vi "Main DAQ Control.vi"() -> ()   [LabVIEW 2012]
uses:
  XControl.xctl
  <vilib>/UeiDaq/UeiDaqCreateDOSession.vi
  <vilib>/UeiDaq/UeiDaqConfigureTimingForSimpleIO.vi
  <vilib>/UeiDaq/UeiDaqWriteOneDigitalScanUInt16.vi
  <vilib>/UeiDaq/UeiDaqWriteDigitalDataUInt16.vi
  <resource>/objmgr/UeiDaq.rc
panel:
  out "Status Indicator":bool[][](array[boolean])
  out "Total Step":u64
  in  "Original Timing Signal (Timing Sequence from Timing File, adjustable on spot)":i16[][](array[numeric])=[[0, 0, 0, 0, 0, 0, 0, 0, 0, 0, 0, 0, 0, 0, 0, 0, 0, 0, 0, 0]] format="%b"
  in  "Digital Output Group 8":T1(xcontrol)
  in  "Digital Output Group 7":T1(xcontrol)
  in  "Group 6":T1(xcontrol)
  in  "Group 5":T1(xcontrol)
  in  "Group 4":T1(xcontrol)
  in  "Group 3":T1(xcontrol)
  in  "Group 2":T1(xcontrol)
  in  "Digital Output Group 1":T1(xcontrol) caption="Group 1"
  out "Running":bool
  in  "DIO Port":string="pwrdaq://Dev0/Do0:2"
  in  "stop":bool
  out "Loop Count":i32
  in  "Loop":bool
  out "Parsed File Location":path
  in  "All Low":bool
  in  "Run":bool
  in  "Timing Array":i32[](array[numeric])=[0, 0, 0, 0, 0, 0, 0, 0, 0, 0, 0, 0, 0, 0, 0, 0, 0, 0, 0, 0] caption="Timing Array (Time Duration for each signal)"
  out "Modified Timing Signal":u16[][](array[numeric]) caption="Modified Timing Signal (after adjustment from I/O channel panel)" format="%b"
  in  "Compile":bool
  in  "GPIB 2":string
  in  "GPIB 1":string
  out "Channel Names":string[](array[string])
  in  "Channel Number":u16
  in  "Load":bool
  in  "Timing File":path
  in  "Perl Parser":path=path "C:/Labview/Parser File/parse-timing.pl"
  # "(Use Do0:5 for DIO0-DIO5, 6ch,  Do0;5 for DIO0 and DIO5, 2ch)"
  # "Control Panel"
  # "(pwrdaq://Dev0 for real I/O; simu://Dev2 for simulated DAQ card)"
  # "I/O Channel"
  # "1"
  # "2"
  # "3"
  # "4"
  # "5"
  # "6"
  # "7"
  # "8"
  # "9"
  # "10"
  # "11"
  # "12"
  # "13"
  # "14"
  # "15"
  # "16"
  # "1"
  # "2"
  # "Group1"
  # "3"
  # "Group2"
  # "4"
  # "Group3"
  # "5"
  # "Group4"
  # "6"
  # "7"
  # "Group5"
  # "8"
  # "Group6"
  # "(Currently, When \"STOP\" is pressed, the status remain in the final state)"
  # "Status Panel"
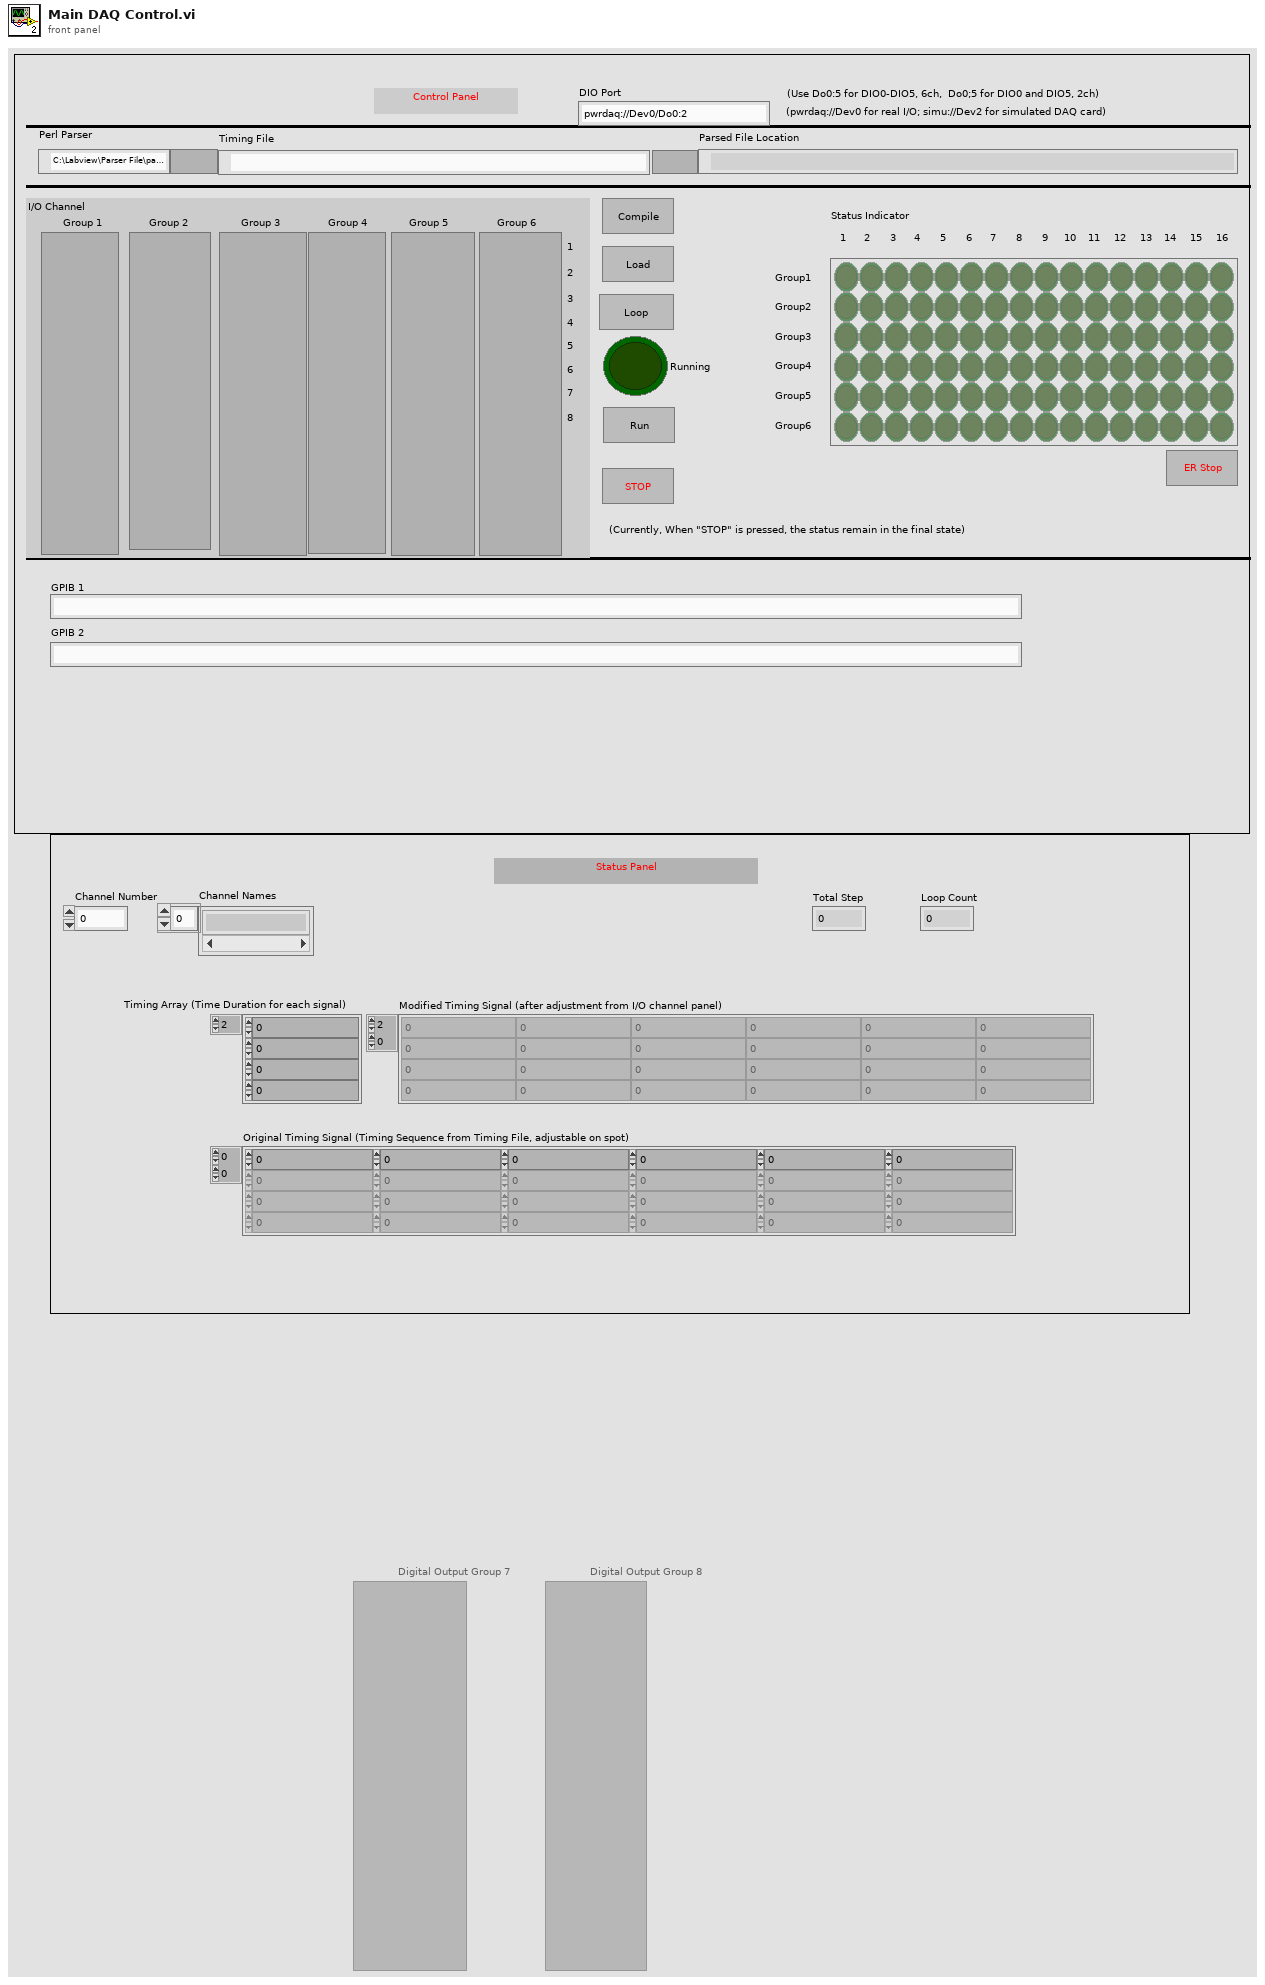
[diagram p1: front panel]
types:
  T1 = cluster{"Channel 1":u8, "Enable":bool, "Main Switch":u8, "Channel 2":u8, "Channel 3":u8, "Channel 4":u8, "Channel 1":u8, "Channel 5":u8, "Channel 6":u8, "Channel 7":u8, "Channel 8":u8, "Channel 9":u8, "Channel 10":u8, "Channel 11":u8, "Channel 1":u8, "Channel 12":u8, "Channel 13":u8, "Channel 14":u8}
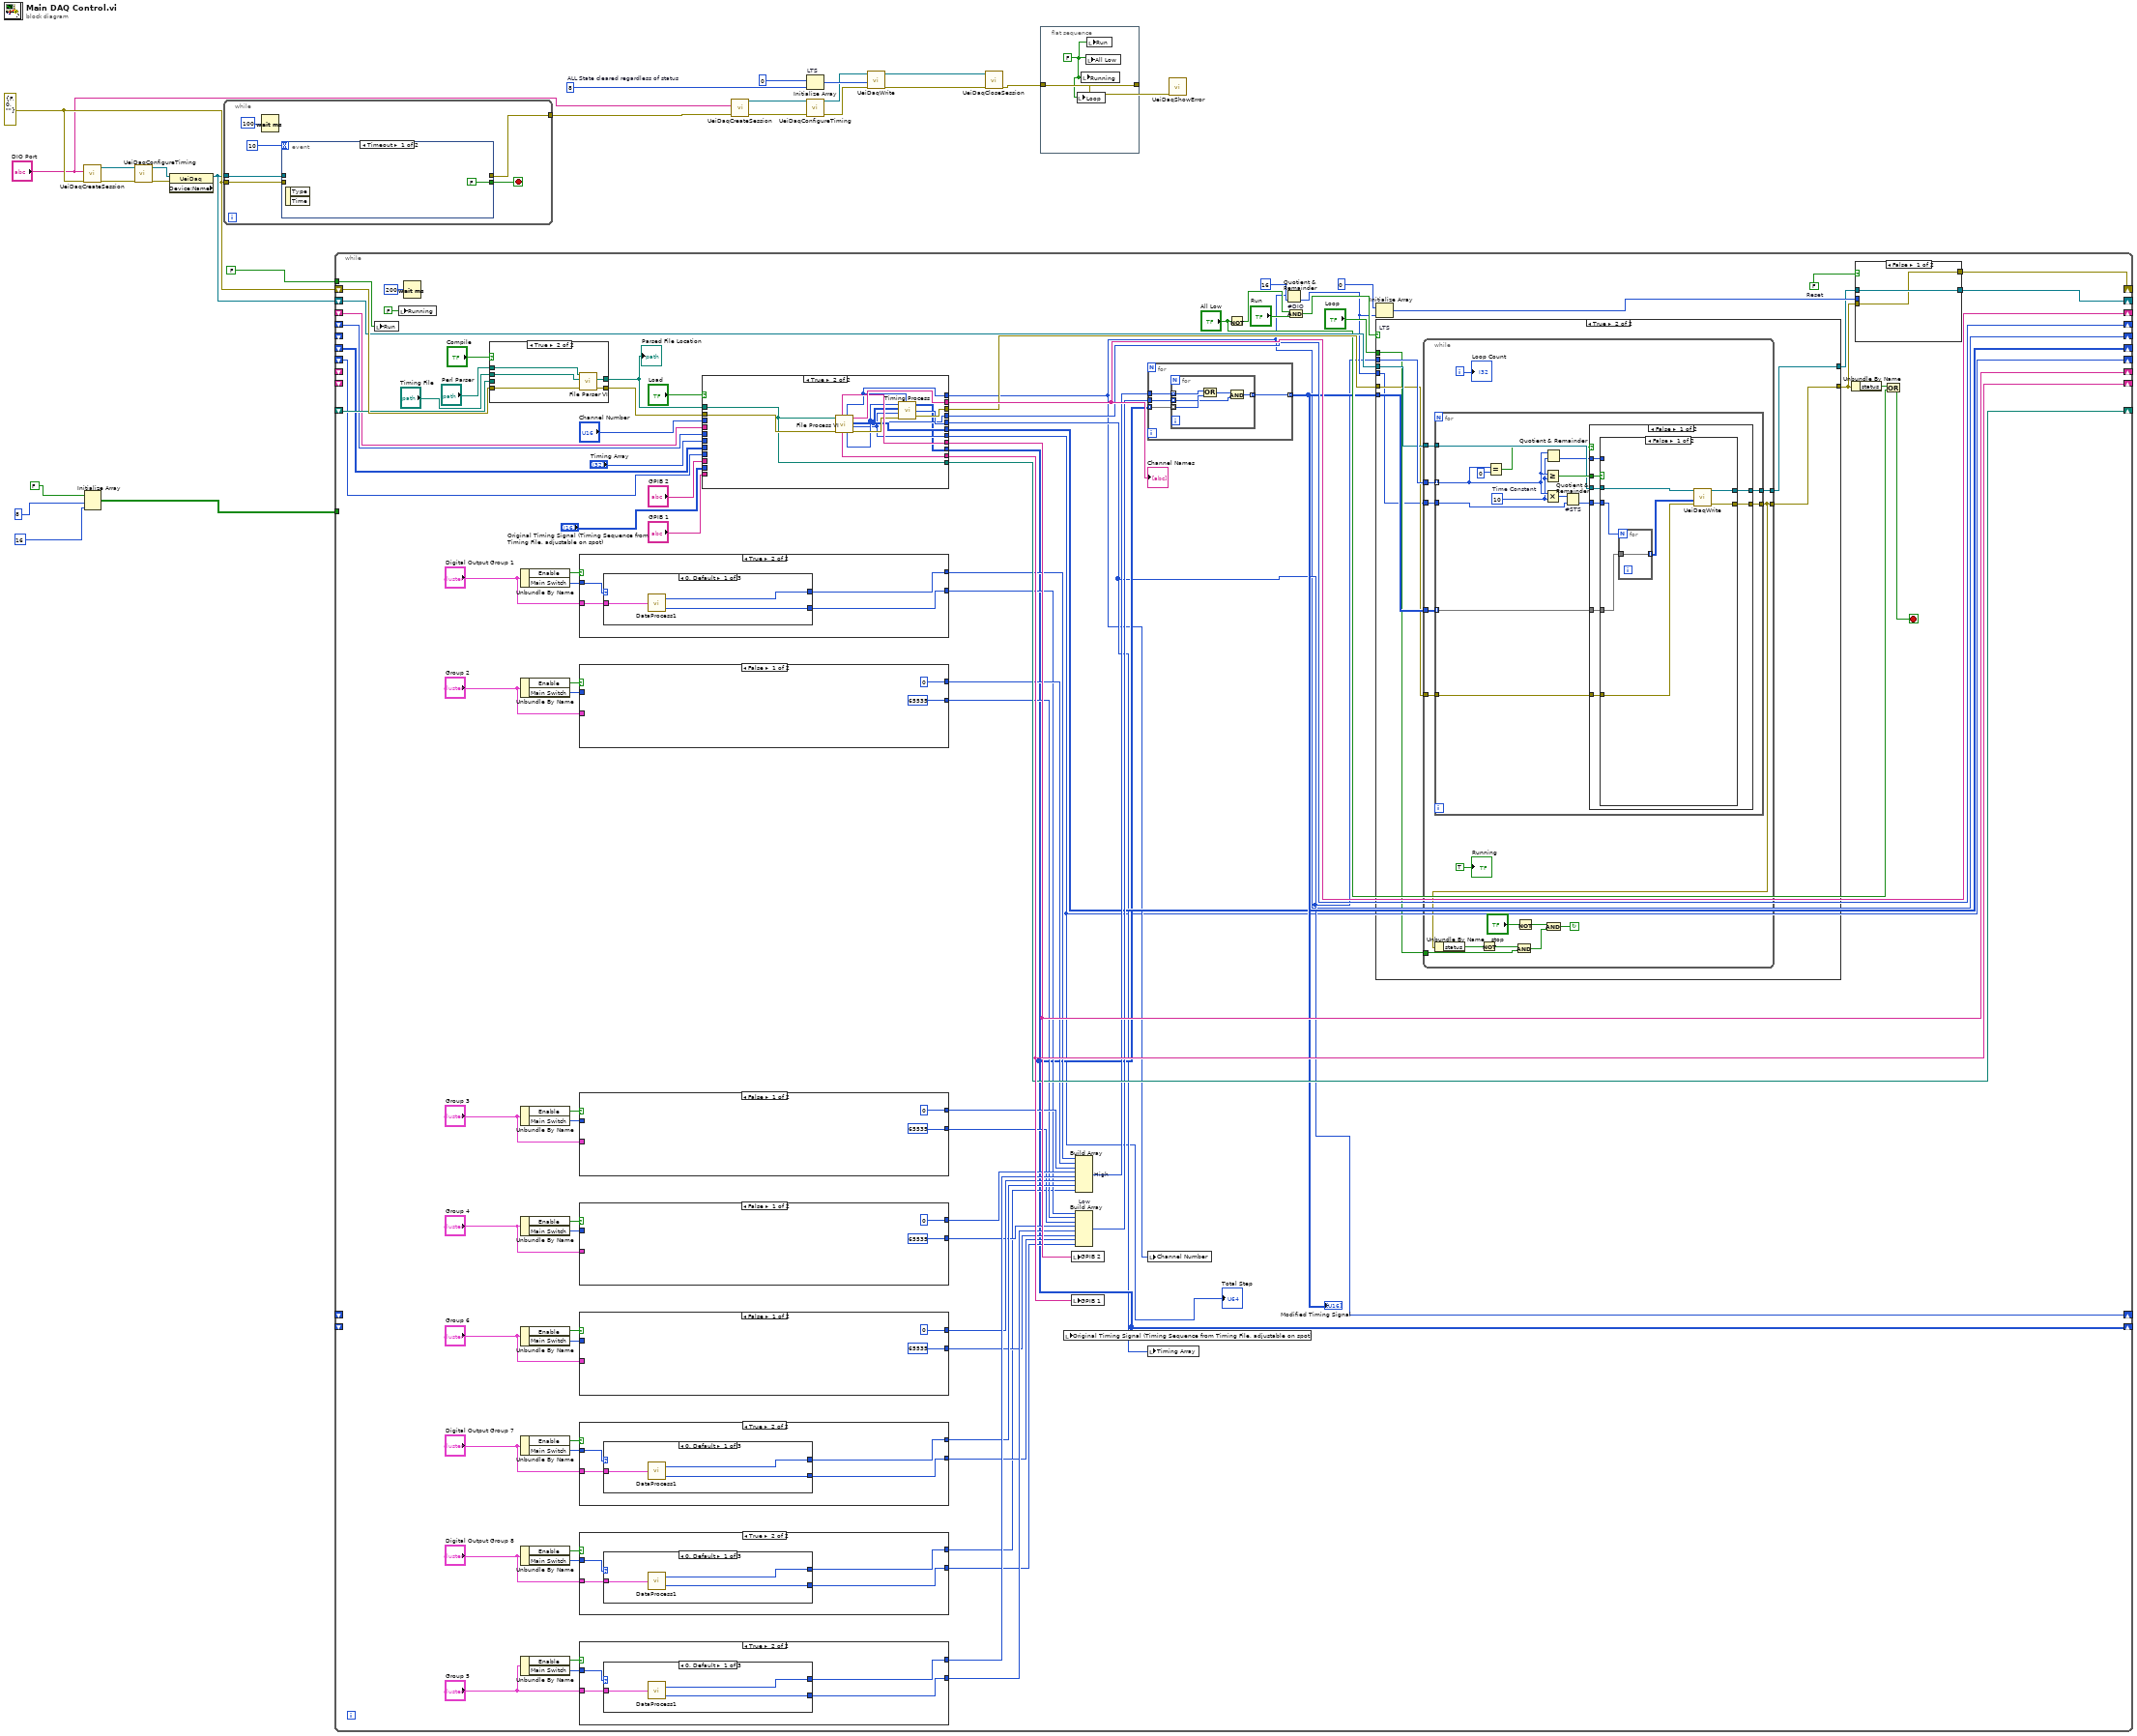
[diagram p0: block diagram]
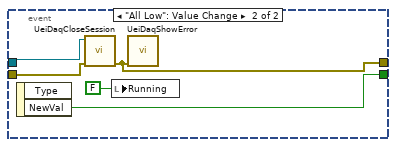
[diagram p2: hidden frame]
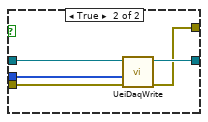
[diagram p3: hidden frame]
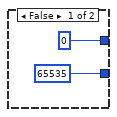
[diagram p4: hidden frame]
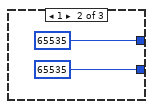
[diagram p5: hidden frame]
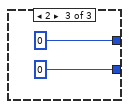
[diagram p6: hidden frame]
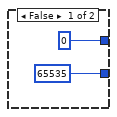
[diagram p7: hidden frame]
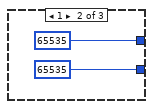
[diagram p8: hidden frame]
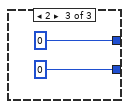
[diagram p9: hidden frame]
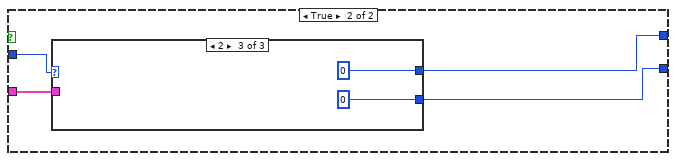
[diagram p10: hidden frame]
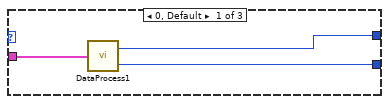
[diagram p11: hidden frame]
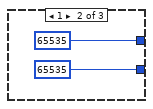
[diagram p12: hidden frame]
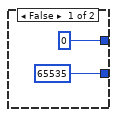
[diagram p13: hidden frame]
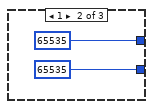
[diagram p14: hidden frame]
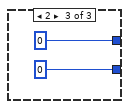
[diagram p15: hidden frame]
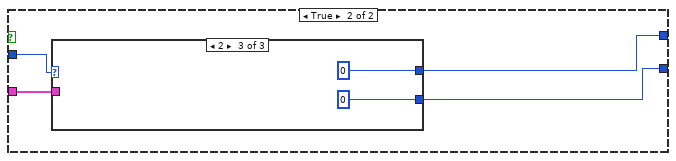
[diagram p16: hidden frame]
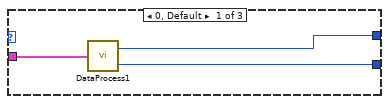
[diagram p17: hidden frame]
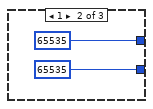
[diagram p18: hidden frame]
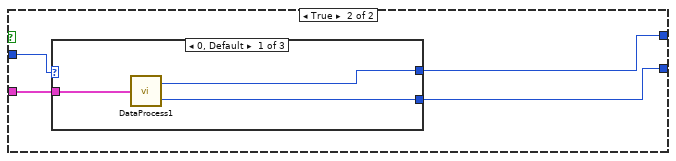
[diagram p19: hidden frame]
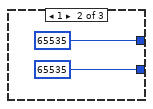
[diagram p20: hidden frame]
diagram:
  w17 = 8  # ALL State cleared regardless of status
  w15 = errorcluster {"status"=FALSE, "code"=0, "source"=""} ("error constant")
  n1 = call-poly <vilib>:"UeiDaqCreateSession.vi"("error in (no error)"=w15, "Resource"="DIO Port") -> ("error out"=w23:errorcluster, "UeiDaq Refnum Out"=w24:refnum<k20>)  [unwired: 8 in]
  n2 = Initialize Array(FALSE, 8, 16) -> (w1:bool[][])
  n3 = call-poly <vilib>:"UeiDaqConfigureTiming.vi"("error in (no error)"=w23, "UeiDaq Refnum In"=w24) -> ("error out"=w21:errorcluster, "UeiDaq Refnum Out"=w22:refnum<k20>)  [unwired: 8 in]
  n4 = property class="UeiDaq" props=["Device:Name"](reference=w22, error in=w21) -> (reference out=w14:refnum<k20>)  [unwired: 2 out]
  n5 = while {
    tunnel: [w29] -> w10
    tunnel: w15 -> [w28]
    tunnel: w14 -> [w27]
    stop <- w30 stop-if-true
    n6 = Wait (ms)(milliseconds to wait=100) -> ()  [unwired: 1 out]
    n7 = event shown="[0] Timeout" {
      selector: _ -> [_ _]
      dyn-events: _ -> [_ _]
      timeout: 10 -> [_ _]
      tunnel: [FALSE w36] -> w30
      tunnel: [_ w33] -> w29
      tunnel: w28 -> [_ w34]
      tunnel: w27 -> [_ w35]
      event Timeout {
        n8 = event-data() -> ()  [unwired: 1 in, 2 out]
      }
      event "All Low": Value Change {
        n9 = event-data() -> ("NewVal"=w36:bool)  [unwired: 1 in, 1 out]
        n10 = call <vilib>:"UeiDaqCloseSession.vi"("error in (no error)"=w34, "UeiDaq Refnum In"=w35) -> ("error out"=w33:errorcluster)  [unwired: 8 in, 1 out]
        n11 = local write "Running"(FALSE) -> ()
        n12 = call <vilib>:"UeiDaqShowError.vi"("error in (no error)"=w33) -> ()  [unwired: 10 in, 1 out]
      }
    }
  }
  n13 = while {
    shift-right: [w99] -> _
    shift-left: w15 -> [w123]
    shift-right: [w112] -> _
    shift-left: _ -> [w122]
    shift-right: [w41] -> _
    shift-left: _ -> [_]
    shift-right: [w120] -> _
    shift-left: _ -> [w121]
    shift-right: [w118] -> _
    shift-left: _ -> [w119]
    shift-right: [w49] -> _
    shift-left: _ -> [w117]
    shift-right: [w116] -> _
    shift-left: _ -> [_]
    shift-right: [w115] -> _
    shift-left: _ -> [_]
    shift-right: [w38] -> _
    shift-left: _ -> [w39]
    shift-right: [w47] -> _
    shift-left: _ -> [_]
    shift-right: [w101] -> _
    shift-left: w14 -> [w110]
    tunnel: FALSE -> [w109]
    shift-right: [w48] -> _
    shift-left: _ -> [_]
    tunnel: w1 -> [_]
    stop <- w105 stop-if-true
    w37 = FALSE  # Reset
    n14 = local write "Run"(w109) -> ()
    n15 = local write "Running"(FALSE) -> ()
    n16 = Wait (ms)(milliseconds to wait=200) -> ()  [unwired: 1 out]
    n17 = case shown="True" "Compile" {
      tunnel: "Timing File" -> [_ w347]
      tunnel: "Perl Parser" -> [_ w346]
      tunnel: [w341 w345] -> w108
      tunnel: [w342 w344] -> w124
      tunnel: w123 -> [w342 w343]
      tunnel: w122 -> [w341 _]
      frame False {
        n18 = Wait (ms)(milliseconds to wait=10) -> ()  [unwired: 1 out]
      }
      frame True {
        n19 = call "File Parser VI.vi"("error in (no error)"=w343, "Original Timing File Path"=w347, "Perl Parser Path"=w346) -> ("error out"=w344:errorcluster, "Parsed File Path"=w345:path)  [unwired: 6 in, 1 out]
      }
    }
    "Parsed File Location" <- w108
    n20 = Unbundle By Name("Digital Output Group 1") -> ("Enable"=w92:bool, "Main Switch"=w91:u8)
    n21 = Unbundle By Name("Group 2") -> ("Enable"=w89:bool, "Main Switch"=w88:u8)
    n22 = Unbundle By Name("Group 3") -> ("Enable"=w86:bool, "Main Switch"=w85:u8)
    n23 = Unbundle By Name("Group 4") -> ("Enable"=w83:bool, "Main Switch"=w82:u8)
    n24 = Unbundle By Name("Group 6") -> ("Enable"=w77:bool, "Main Switch"=w76:u8)
    n25 = Unbundle By Name("Digital Output Group 7") -> ("Enable"=w74:bool, "Main Switch"=w73:u8)
    n26 = Unbundle By Name("Digital Output Group 8") -> ("Enable"=w71:bool, "Main Switch"=w70:u8)
    n27 = Unbundle By Name("Group 5") -> ("Enable"=w80:bool, "Main Switch"=w79:u8)
    n28 = case shown="True" w92 {
      tunnel: [u16 0 w238] -> w68
      tunnel: [u16 65535 w237] -> w61
      tunnel: w91 -> [_ w240]
      tunnel: "Digital Output Group 1" -> [_ w239]
      frame False {
      }
      frame True {
        n29 = case shown="0, Default" w240 {
          tunnel: w239 -> [w241 _ _]
          tunnel: [w243 u16 65535 u16 0] -> w238
          tunnel: [w242 u16 65535 u16 0] -> w237
          frame 0, Default {
            n30 = call "DataProcess1.vi"("XControl"=w241) -> ("High Out"=w243:u16, "Low Out"=w242:u16)
          }
          frame 1 {
          }
          frame 2 {
          }
        }
      }
    }
    n31 = case shown="False" w89 {
      tunnel: [u16 0 w225] -> w67
      tunnel: [u16 65535 w224] -> w60
      tunnel: w88 -> [_ w227]
      tunnel: "Group 2" -> [_ w226]
      frame False {
      }
      frame True {
        n32 = case shown="2" w227 {
          tunnel: w226 -> [w230 _ _]
          tunnel: [w229 u16 65535 u16 0] -> w225
          tunnel: [w228 u16 65535 u16 0] -> w224
          frame 0, Default {
            n33 = call "DataProcess1.vi"("XControl"=w230) -> ("High Out"=w229:u16, "Low Out"=w228:u16)
          }
          frame 1 {
          }
          frame 2 {
          }
        }
      }
    }
    n34 = case shown="False" w86 {
      tunnel: [u16 0 w212] -> w66
      tunnel: [u16 65535 w211] -> w59
      tunnel: w85 -> [_ w214]
      tunnel: "Group 3" -> [_ w213]
      frame False {
      }
      frame True {
        n35 = case shown="0, Default" w214 {
          tunnel: w213 -> [w217 _ _]
          tunnel: [w216 u16 65535 u16 0] -> w212
          tunnel: [w215 u16 65535 u16 0] -> w211
          frame 0, Default {
            n36 = call "DataProcess1.vi"("XControl"=w217) -> ("High Out"=w216:u16, "Low Out"=w215:u16)
          }
          frame 1 {
          }
          frame 2 {
          }
        }
      }
    }
    n37 = case shown="False" w83 {
      tunnel: [u16 0 w199] -> w65
      tunnel: [u16 65535 w198] -> w58
      tunnel: w82 -> [_ w201]
      tunnel: "Group 4" -> [_ w200]
      frame False {
      }
      frame True {
        n38 = case shown="2" w201 {
          tunnel: w200 -> [w204 _ _]
          tunnel: [w203 u16 65535 u16 0] -> w199
          tunnel: [w202 u16 65535 u16 0] -> w198
          frame 0, Default {
            n39 = call "DataProcess1.vi"("XControl"=w204) -> ("High Out"=w203:u16, "Low Out"=w202:u16)
          }
          frame 1 {
          }
          frame 2 {
          }
        }
      }
    }
    n40 = case shown="False" w77 {
      tunnel: [u16 0 w173] -> w63
      tunnel: [u16 65535 w172] -> w56
      tunnel: w76 -> [_ w175]
      tunnel: "Group 6" -> [_ w174]
      frame False {
      }
      frame True {
        n41 = case shown="2" w175 {
          tunnel: w174 -> [w178 _ _]
          tunnel: [w177 u16 65535 u16 0] -> w173
          tunnel: [w176 u16 65535 u16 0] -> w172
          frame 0, Default {
            n42 = call "DataProcess1.vi"("XControl"=w178) -> ("High Out"=w177:u16, "Low Out"=w176:u16)
          }
          frame 1 {
          }
          frame 2 {
          }
        }
      }
    }
    n43 = case shown="True" w74 {
      tunnel: [u16 0 w160] -> w62
      tunnel: [u16 65535 w159] -> w55
      tunnel: w73 -> [_ w162]
      tunnel: "Digital Output Group 7" -> [_ w161]
      frame False {
      }
      frame True {
        n44 = case shown="0, Default" w162 {
          tunnel: w161 -> [w165 _ _]
          tunnel: [w164 u16 65535 u16 0] -> w160
          tunnel: [w163 u16 65535 u16 0] -> w159
          frame 0, Default {
            n45 = call "DataProcess1.vi"("XControl"=w165) -> ("High Out"=w164:u16, "Low Out"=w163:u16)
          }
          frame 1 {
          }
          frame 2 {
          }
        }
      }
    }
    n46 = case shown="True" w71 {
      tunnel: [u16 0 w147] -> w54
      tunnel: [u16 65535 w146] -> w53
      tunnel: w70 -> [_ w149]
      tunnel: "Digital Output Group 8" -> [_ w148]
      frame False {
      }
      frame True {
        n47 = case shown="0, Default" w149 {
          tunnel: w148 -> [w152 _ _]
          tunnel: [w151 u16 65535 u16 0] -> w147
          tunnel: [w150 u16 65535 u16 0] -> w146
          frame 0, Default {
            n48 = call "DataProcess1.vi"("XControl"=w152) -> ("High Out"=w151:u16, "Low Out"=w150:u16)
          }
          frame 1 {
          }
          frame 2 {
          }
        }
      }
    }
    n49 = case shown="True" w80 {
      tunnel: [u16 0 w186] -> w64
      tunnel: [u16 65535 w185] -> w57
      tunnel: w79 -> [_ w188]
      tunnel: "Group 5" -> [_ w187]
      frame False {
      }
      frame True {
        n50 = case shown="0, Default" w188 {
          tunnel: w187 -> [w191 _ _]
          tunnel: [w190 u16 65535 u16 0] -> w186
          tunnel: [w189 u16 65535 u16 0] -> w185
          frame 0, Default {
            n51 = call "DataProcess1.vi"("XControl"=w191) -> ("High Out"=w190:u16, "Low Out"=w189:u16)
          }
          frame 1 {
          }
          frame 2 {
          }
        }
      }
    }
    n52 = case shown="True" "Load" {
      tunnel: w108 -> [w325 w335]
      tunnel: w124 -> [w326 w339]
      tunnel: [w321 w330] -> w49
      tunnel: [w322 w329] -> w118
      tunnel: [w324 w334] -> w41
      tunnel: [w319 w328] -> w38
      tunnel: [w323 w338] -> w120
      tunnel: [w315 w337] -> w116
      tunnel: [w320 w336] -> w115
      tunnel: [w326 w332] -> w111
      tunnel: [w325 w335] -> w112
      tunnel: "Channel Number" -> [w324 _]
      tunnel: w121 -> [w323 _]
      tunnel: w119 -> [w322 _]
      tunnel: w117 -> [w321 _]
      tunnel: "GPIB 2" -> [w320 _]
      tunnel: w39 -> [w319 _]
      tunnel: [w318 w331] -> w47
      tunnel: "Timing Array" -> [w318 _]
      tunnel: [w316 w327] -> w48
      tunnel: "Original Timing Signal (Timing Sequence from Timing File, adjustable on spot)" -> [w316 _]
      tunnel: "GPIB 1" -> [w315 _]
      frame False {
        n53 = Wait (ms)(milliseconds to wait=10) -> ()  [unwired: 1 out]
      }
      frame True {
        n54 = call "File Process VI.vi"("error in (no error)"=w339, "Parsed File Path"=w335) -> ("Error Out"=w333:errorcluster, "Total Step"=w328:u64, "Switching Times"=w330:u32[][], "Channel Names"=w338:string[], "Initial States"=w329:u16[], "Channel Number"=w334:u16, "GPIB 1"=w337:string, "GPIB 2"=w336:string)  [unwired: 2 in]
        n55 = call "Timing Process.vi"("Initial States"=w329, "Switching Times"=w330, "Total Steps"=w328, "error in (no error)"=w333, "Channel"=w334) -> ("Output Signal Array"=w327:i16[][], "Output Time Array"=w331:i32[], "error out"=w332:errorcluster)
      }
    }
    "Channel Names" <- w120
    "Total Step" <- w38
    n56 = local write "Original Timing Signal (Timing Sequence from Timing File, adjustable on spot)"(w48) -> ()
    n57 = local write "GPIB 2"(w115) -> ()
    n58 = local write "GPIB 1"(w116) -> ()
    n59 = Build Array "High"(w68, w67, w66, w65, w64, w63, w62, w54) -> (w52:u16[])
    n60 = Build Array "Low"(w61, w60, w59, w58, w57, w56, w55, w53) -> (w51:u16[])
    n61 = for {
      tunnel: w48 -> [w138] mode=indexing
      tunnel: w52 -> [w137]
      tunnel: w51 -> [w136]
      tunnel: [w135] -> w50 mode=indexing
      n62 = for {
        tunnel: w138 -> [w143] mode=indexing
        tunnel: w137 -> [w142] mode=indexing
        tunnel: w136 -> [w140] mode=indexing
        tunnel: [w139] -> w135 mode=indexing
        n63 = Or(x=w142, y=w143) -> (x .or. y?=w141:u16)
        n64 = And(x=w141, y=w140) -> (x .and. y?=w139:u16)
      }
    }
    "Modified Timing Signal" <- w50
    n65 = local write "Channel Number"(w41) -> ()
    n66 = local write "Timing Array"(w47) -> ()
    n67 = Not(x="All Low") -> (.not. x?=w95:bool)
    n68 = Quotient & Remainder "#DIO"(x=w41, y=u16 16) -> (floor(x/y)=w93:u16)  [unwired: 1 out]
    n69 = And(x=w95, y="Run") -> (x .and. y?=w96:bool)
    n70 = Initialize Array "LTS"(i16 0, w93) -> (w103:i16[])
    n71 = case shown="True" w96 {
      tunnel: w47 -> [_ w257]
      tunnel: w50 -> [_ w256]
      tunnel: w110 -> [w249 w255]
      tunnel: w111 -> [w248 w254]
      tunnel: "Loop" -> [_ w253]
      tunnel: [w248 w252] -> w100
      tunnel: [w249 w251] -> w102
      tunnel: w93 -> [_ w250]
      frame False {
      }
      frame True {
        n72 = while {
          tunnel: w257 -> [w273]
          tunnel: w256 -> [w272]
          tunnel: w255 -> [w271]
          tunnel: w254 -> [w260]
          tunnel: w253 -> [w268]
          tunnel: [w258] -> w252
          tunnel: [w269] -> w251
          tunnel: w250 -> [w262]
          i -> [w267]
          stop <- w264 continue-if-true
          n73 = for {
            tunnel: w273 -> [w278] mode=indexing
            tunnel: w272 -> [w282] mode=indexing
            tunnel: w271 -> [w286]
            tunnel: w260 -> [w285]
            tunnel: [w284] -> w258
            tunnel: [w281] -> w269
            tunnel: w262 -> [w276]
            w274 = 10  # Time Constant
            n74 = Equal?(x=w278, y=0) -> (x = y?=w279:bool)
            n75 = Greater Or Equal?(x=w278, y=w274) -> (x >= y?=w287:bool)
            n76 = Multiply(x=w278, y=w274) -> (x*y=w277:i32)
            n77 = Quotient & Remainder(x=w278, y=w274) -> (floor(x/y)=w283:i32)  [unwired: 1 out]
            n78 = Quotient & Remainder "#STS"(x=w277, y=w276) -> (floor(x/y)=w275:i32)  [unwired: 1 out]
            n79 = case shown="False" w279 {
              tunnel: w287 -> [w295 _]
              tunnel: w286 -> [w294 w314]
              tunnel: w285 -> [w293 w313]
              tunnel: [w292 w313] -> w284
              tunnel: w283 -> [w291 _]
              tunnel: w282 -> [w290 _]
              tunnel: [w289 w314] -> w281
              tunnel: w275 -> [w288 _]
              frame False {
                n80 = case shown="False" w295 {
                  tunnel: w294 -> [w300 w310]
                  tunnel: w293 -> [w302 w309]
                  tunnel: [w301 w308] -> w292
                  tunnel: w291 -> [_ w307]
                  tunnel: w290 -> [w296 w305]
                  tunnel: [w299 w306] -> w289
                  tunnel: w288 -> [w298 _]
                  frame False {
                    n81 = for {
                      N: w298 -> [_]
                      tunnel: [w303] -> w297 mode=indexing
                      tunnel: w296 -> [w303]
                    }
                    n82 = call-poly <vilib>:"UeiDaqWrite.vi"("error in (no error)"=w302, "Digital Data"=w297, "UeiDaq Refnum In"=w300) -> ("error out"=w301:errorcluster, "UeiDaq Refnum Out"=w299:refnum<k20>)  [unwired: 7 in]
                  }
                  frame True {
                    n83 = Wait (ms)(milliseconds to wait=w307) -> ()  [unwired: 1 out]
                    n84 = for {
                      tunnel: w305 -> [w312] mode=indexing
                      tunnel: [w311] -> w304 mode=indexing
                      n85 = Number To Boolean Array(number=w312) -> (Boolean array=w311:bool[])
                    }
                    "Status Indicator" <- w304
                    n86 = call-poly <vilib>:"UeiDaqWrite.vi"("error in (no error)"=w309, "Digital Data"=w305, "UeiDaq Refnum In"=w310) -> ("error out"=w308:errorcluster, "UeiDaq Refnum Out"=w306:refnum<k20>)  [unwired: 7 in]
                  }
                }
              }
              frame True {
              }
            }
          }
          n87 = Unbundle By Name(w258) -> ("status"=w259:bool)
          n88 = Not(x=w259) -> (.not. x?=w270:bool)
          n89 = And(x=w270, y=w268) -> (x .and. y?=w266:bool)
          n90 = Not(x="stop") -> (.not. x?=w263:bool)
          n91 = And(x=w263, y=w266) -> (x .and. y?=w264:bool)
          "Loop Count" <- w267
          "Running" <- TRUE
        }
      }
    }
    n92 = Unbundle By Name(w100) -> ("status"=w106:bool)
    n93 = case shown="False" w37 {
      tunnel: w103 -> [_ w134]
      tunnel: w102 -> [w129 w133]
      tunnel: [w129 w132] -> w101
      tunnel: w100 -> [w128 w131]
      tunnel: [w128 w130] -> w99
      frame False {
      }
      frame True {
        n94 = call-poly <vilib>:"UeiDaqWrite.vi"("error in (no error)"=w131, "Digital Data"=w134, "UeiDaq Refnum In"=w133) -> ("error out"=w130:errorcluster, "UeiDaq Refnum Out"=w132:refnum<k20>)  [unwired: 7 in]
      }
    }
    n95 = Or(x=w106, y="All Low") -> (x .or. y?=w105:bool)
  }
  n96 = call-poly <vilib>:"UeiDaqCreateSession.vi"("error in (no error)"=w10, "Resource"="DIO Port") -> ("error out"=w11:errorcluster, "UeiDaq Refnum Out"=w12:refnum<k20>)  [unwired: 8 in]
  n97 = Initialize Array "LTS"(i16 0, w17) -> (w16:i16[])
  n98 = call-poly <vilib>:"UeiDaqConfigureTiming.vi"("error in (no error)"=w11, "UeiDaq Refnum In"=w12) -> ("error out"=w8:errorcluster, "UeiDaq Refnum Out"=w9:refnum<k20>)  [unwired: 8 in]
  n99 = call-poly <vilib>:"UeiDaqWrite.vi"("error in (no error)"=w8, "Digital Data"=w16, "UeiDaq Refnum In"=w9) -> ("error out"=w19:errorcluster, "UeiDaq Refnum Out"=w20:refnum<k20>)  [unwired: 7 in]
  n100 = call <vilib>:"UeiDaqCloseSession.vi"("error in (no error)"=w19, "UeiDaq Refnum In"=w20) -> ("error out"=w5:errorcluster)  [unwired: 8 in, 1 out]
  n101 = flat-sequence {
    tunnel: [w349] -> w6
    tunnel: w5 -> [w349]
    frame #0 {
      w348 = FALSE
      n102 = local write "Loop"(w348) -> ()
      n103 = local write "Running"(w348) -> ()
      n104 = local write "All Low"(w348) -> ()
      n105 = local write "Run"(w348) -> ()
    }
  }
  n106 = call <vilib>:"UeiDaqShowError.vi"("error in (no error)"=w6) -> ()  [unwired: 10 in, 1 out]
